vi "GDSString_FromatedTextToHTML.vi"(8 "error in (no error)":errorcluster, 11 "FormattedStringIn":refnum<vi>) -> (0 "error out":errorcluster, 2 "TextOut":string="<B</<1700FF<I</000000</I>>>>B>>ABCD", 3 "FormattedStringOut":refnum<vi>)   [LabVIEW 2020]
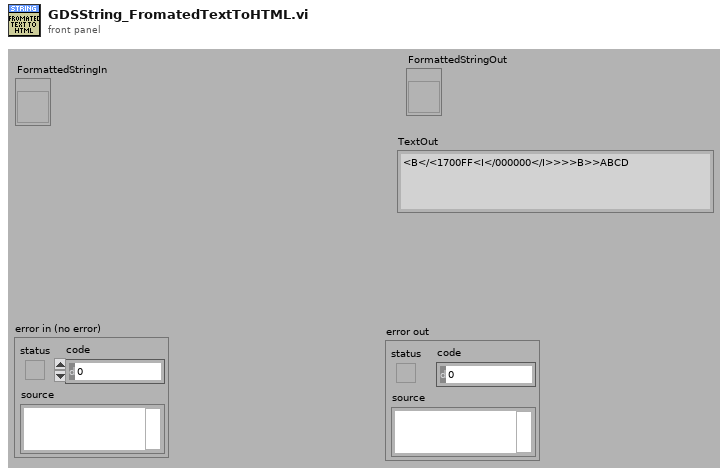
[diagram p1: front panel]
types:
  T1 = cluster{"i":i32, "Start":bool, "Type":enum16{"B", "I", "U", "C"}, "Data":variant}[]
  T2 = cluster{"i":i32, "Start":bool, "Type":enum16{"B", "I", "U", "C"}, "Data":variant}
  T3 = typedef "LVFontTypeDef.ctl" = cluster{"Font Name":string, "Size":u16, "Bold":bool, "Italic":bool, "Underline":bool, "Strikeout":bool, "Color":u32}
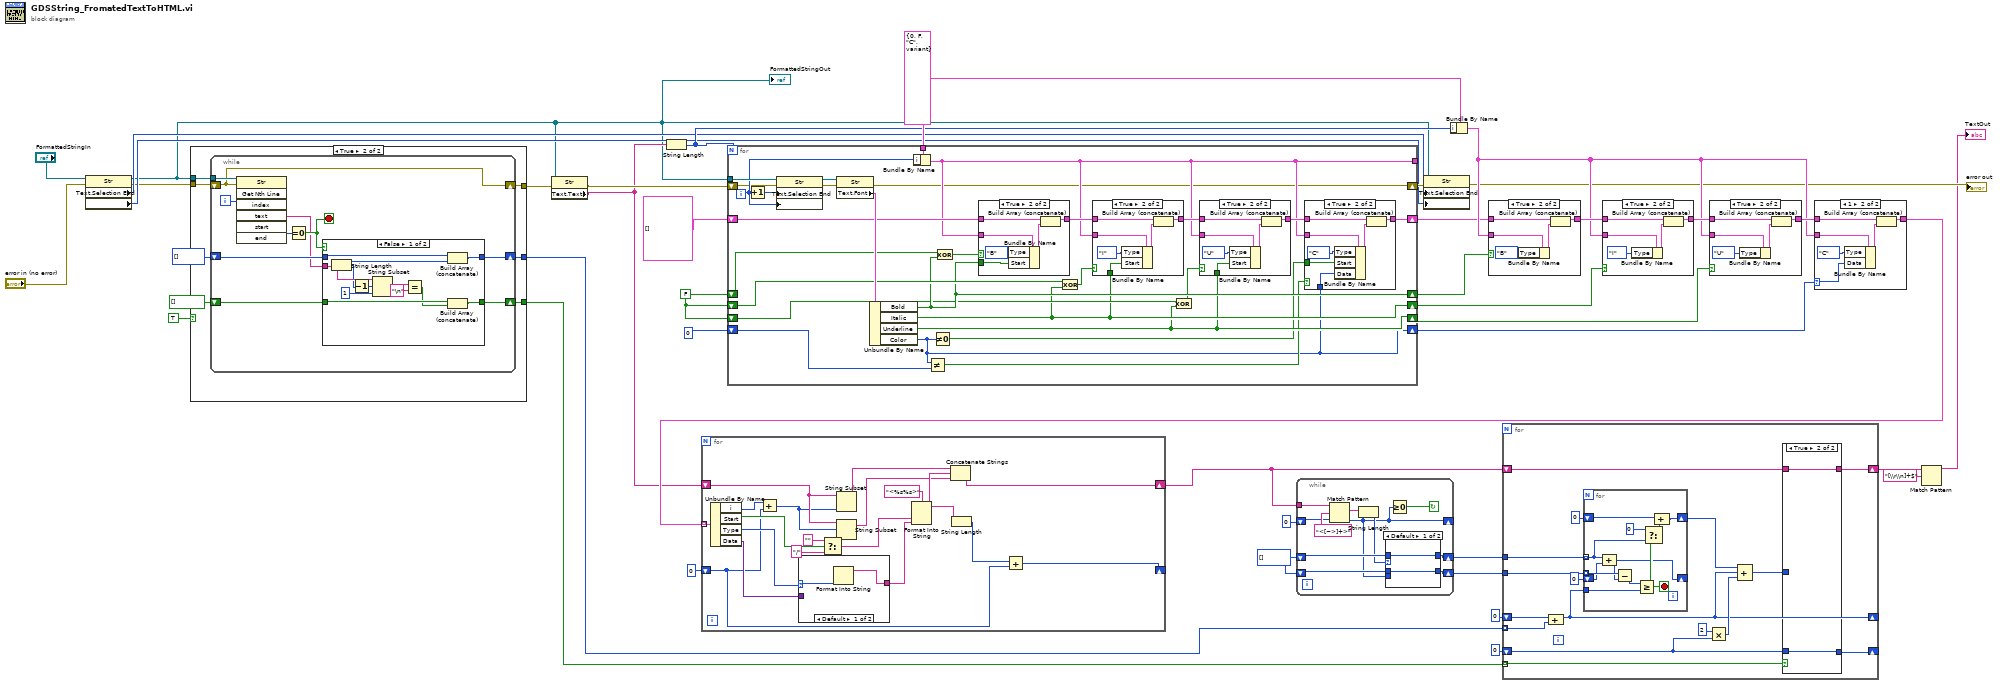
[diagram p0: block diagram]
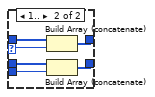
[diagram p2: hidden frame]
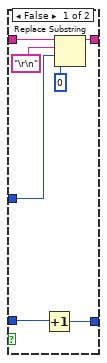
[diagram p3: hidden frame]
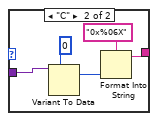
[diagram p10: hidden frame]
diagram:
  w11 = i32[] []
  w39 = FALSE ("Bold")
  w30 = T2 {"i"=0, "Start"=FALSE, "Type"=enum."C", "Data"=variant}
  n1 = property on="Property Node" class="Str"(reference="FormattedStringIn", error in="error in (no error)") -> (reference out=w13:refnum<vi>, error out=w17:errorcluster, "Text.Selection End"=w20:u32, "Text.Selection Start"=w19:u32)
  "FormattedStringOut" <- w13
  n2 = case shown="True" TRUE {
    tunnel: w13 -> [_ w48]
    tunnel: w17 -> [w41 w47]
    tunnel: [_ w45] -> w6
    tunnel: [w41 w46] -> w16
    tunnel: [_ w42] -> w2
    frame False {
    }
    frame True {
      n3 = while {
        tunnel: w48 -> [w57]
        shift-right: [w55] -> w45
        shift-left: i32[] [] -> [w54]
        shift-right: [w53] -> w46
        shift-left: w47 -> [w53]
        shift-right: [w51] -> w42
        shift-left: bool[] [] -> [w52]
        i -> [w58]
        stop <- w56 stop-if-true
        n4 = invoke on="Invoke Node" class="Str" method="Get Nth Line"(reference=w57, error in=w53, "index"=w58) -> ("text"=w50:string, "end"=w49:u32)  [unwired: 4 in, 5 out]
        n5 = Equal To 0?(x=w49) -> (x = 0?=w56:bool)
        n6 = case shown="False" w56 {
          tunnel: w50 -> [w65 _]
          tunnel: [w68 w71] -> w55
          tunnel: w54 -> [w69 w71]
          tunnel: [w67 w70] -> w51
          tunnel: w52 -> [w66 w70]
          frame False {
            n7 = String Length(string=w65) -> (length=w60:i32)
            n8 = Decrement(x=w60) -> (x-1=w63:i32)
            n9 = String Subset(string=w65, offset (0)=w63, length (rest)=1 ("length (rest)")) -> (substring=w62:string)
            n10 = Equal?(x=w62, y="\n") -> (x = y?=w59:bool)
            n11 = Build Array (concatenate)(w69, w60) -> (w68:i32[])
            n12 = Build Array (concatenate)(w66, w59) -> (w67:bool[])
          }
          frame True {
          }
        }
      }
    }
  }
  n13 = property class="Str"(reference=w13, error in=w16) -> (error out=w15:errorcluster, "Text.Text"=w14:string)  [unwired: 1 out]
  n14 = String Length(string=w14) -> (length=w29:i32)
  n15 = for {
    N: w29 -> [_]
    tunnel: w13 -> [w99]
    shift-right: [w90] -> w27
    shift-left: T1 [] -> [w95]
    tunnel: w30 -> [w94]
    shift-right: [w84] -> w34
    shift-left: w39 -> [w88]
    shift-right: [w81] -> w33
    shift-left: w39 -> [w85]
    shift-right: [w80] -> w32
    shift-left: w39 -> [w82]
    shift-right: [w76] -> w31
    shift-left: u32 0 ("Color") -> [w79]
    tunnel: [w75] -> _
    shift-right: [w72] -> w22
    shift-left: w15 -> [w74]
    i -> [w93]
    n16 = Increment(x=w93) -> (x+1=w97:i32)
    n17 = property class="Str"(reference=w99, error in=w74, "Text.Selection End"=w97, "Text.Selection Start"=w93) -> (reference out=w98:refnum<vi>, error out=w73:errorcluster)
    n18 = property class="Str"(reference=w98, error in=w73) -> (error out=w72:errorcluster, "Text.Font"=w96:T3)  [unwired: 1 out]
    n19 = Unbundle By Name(w96) -> ("Bold"=w84:bool, "Italic"=w81:bool, "Underline"=w80:bool, "Color"=w76:u32)
    n20 = Bundle By Name(cluster=w94, "i"=w93) -> (w75:T2)
    n21 = Not Equal?(x=w76, y=w79) -> (x != y?=w78:bool)
    n22 = Not Equal To 0?(x=w76) -> (x != 0?=w77:bool)
    n23 = Exclusive Or(1:w84, 2:w88) -> (0:w87:bool)
    n24 = case shown="True" w87 {
      tunnel: w95 -> [w122 w128]
      tunnel: [w122 w127] -> w92
      tunnel: w75 -> [_ w126]
      tunnel: w84 -> [_ w123]
      frame False {
      }
      frame True {
        n25 = Bundle By Name(cluster=w126, "Type"=enum16{"B", "I", "U", "C"}."B", "Start"=w123) -> (w125:T2)
        n26 = Build Array (concatenate)(w128, w125) -> (w127:T1)
      }
    }
    n27 = Exclusive Or(1:w81, 2:w85) -> (0:w86:bool)
    n28 = case shown="True" w86 {
      tunnel: w92 -> [w115 w121]
      tunnel: [w115 w120] -> w91
      tunnel: w75 -> [_ w119]
      tunnel: w81 -> [_ w116]
      frame False {
      }
      frame True {
        n29 = Bundle By Name(cluster=w119, "Type"=enum16{"B", "I", "U", "C"}."I", "Start"=w116) -> (w118:T2)
        n30 = Build Array (concatenate)(w121, w118) -> (w120:T1)
      }
    }
    n31 = Exclusive Or(1:w80, 2:w82) -> (0:w83:bool)
    n32 = case shown="True" w83 {
      tunnel: w91 -> [w108 w114]
      tunnel: [w108 w113] -> w89
      tunnel: w75 -> [_ w112]
      tunnel: w80 -> [_ w109]
      frame False {
      }
      frame True {
        n33 = Bundle By Name(cluster=w112, "Type"=enum16{"B", "I", "U", "C"}."U", "Start"=w109) -> (w111:T2)
        n34 = Build Array (concatenate)(w114, w111) -> (w113:T1)
      }
    }
    n35 = case shown="True" w78 {
      tunnel: w89 -> [w100 w107]
      tunnel: [w100 w106] -> w90
      tunnel: w75 -> [_ w105]
      tunnel: w76 -> [_ w102]
      tunnel: w77 -> [_ w101]
      frame False {
      }
      frame True {
        n36 = Bundle By Name(cluster=w105, "Type"=enum16{"B", "I", "U", "C"}."C", "Start"=w101, "Data"=w102) -> (w104:T2)
        n37 = Build Array (concatenate)(w107, w104) -> (w106:T1)
      }
    }
  }
  n38 = property on="Property Node" class="Str"(reference=w13, error in=w22, "Text.Selection End"=w20, "Text.Selection Start"=w19) -> (error out=→"error out":errorcluster)  [unwired: 1 out]
  n39 = Bundle By Name(cluster=w30, "i"=w29) -> (w28:T2)
  n40 = case shown="True" w34 {
    tunnel: w27 -> [w129 w134]
    tunnel: [w129 w133] -> w35
    tunnel: w28 -> [_ w132]
    frame False {
    }
    frame True {
      n41 = Bundle By Name(cluster=w132, "Type"=enum16{"B", "I", "U", "C"}."B") -> (w131:T2)
      n42 = Build Array (concatenate)(w134, w131) -> (w133:T1)
    }
  }
  n43 = case shown="True" w33 {
    tunnel: w35 -> [w135 w140]
    tunnel: [w135 w139] -> w36
    tunnel: w28 -> [_ w138]
    frame False {
    }
    frame True {
      n44 = Bundle By Name(cluster=w138, "Type"=enum16{"B", "I", "U", "C"}."I") -> (w137:T2)
      n45 = Build Array (concatenate)(w140, w137) -> (w139:T1)
    }
  }
  n46 = case shown="True" w32 {
    tunnel: w36 -> [w141 w146]
    tunnel: [w141 w145] -> w37
    tunnel: w28 -> [_ w144]
    frame False {
    }
    frame True {
      n47 = Bundle By Name(cluster=w144, "Type"=enum16{"B", "I", "U", "C"}."U") -> (w143:T2)
      n48 = Build Array (concatenate)(w146, w143) -> (w145:T1)
    }
  }
  n49 = case shown="1" w31 {
    selector: w31 -> [_ w148]
    tunnel: w37 -> [w147 w153]
    tunnel: [w147 w152] -> w26
    tunnel: w28 -> [_ w151]
    frame 0, Default {
    }
    frame 1 {
      n50 = Bundle By Name(cluster=w151, "Type"=enum16{"B", "I", "U", "C"}."C", "Data"=w148) -> (w150:T2)
      n51 = Build Array (concatenate)(w153, w150) -> (w152:T1)
    }
  }
  n52 = for {
    shift-right: [w155] -> w7
    shift-left: w14 -> [w165]
    tunnel: w26 -> [w172] mode=indexing
    shift-right: [w162] -> _
    shift-left: 0 -> [w160]
    n53 = Unbundle By Name(w172) -> ("i"=w161:i32, "Start"=w170:bool, "Type"=w167:enum16{"B", "I", "U", "C"}, "Data"=w166:variant)
    n54 = Add(x=w161, y=w160) -> (x+y=w159:i32)
    n55 = case shown="Default" w167 {
      selector: w167 -> [w174 _]
      tunnel: [w173 w175] -> w164
      tunnel: w166 -> [_ w179]
      frame Default {
        n56 = Format Into String(w174) -> (resulting string=w173:string)  [unwired: 3 in, 1 out]
      }
      frame "C" {
        n57 = Variant To Data(type=u32 0 ("Color"), Variant=w179) -> (data=w177:u32)  [unwired: 1 in, 1 out]
        n58 = Format Into String(format string="0x%06X", w177) -> (resulting string=w175:string)  [unwired: 2 in, 1 out]
      }
    }
    n59 = Select(t="", s=w170, f="/" ("format string")) -> (s? t:f=w163:string)
    n60 = String Subset(string=w165, length (rest)=w159) -> (substring=w158:string)  [unwired: 1 out]
    n61 = String Subset(string=w165, offset (0)=w159) -> (substring=w156:string)  [unwired: 1 out]
    n62 = Format Into String(format string="<%s%s>", w163, w164) -> (resulting string=w157:string)  [unwired: 2 in, 1 out]
    n63 = Concatenate Strings(w158, w157, w156) -> (w155:string)
    n64 = String Length(string=w157) -> (length=w154:i32)
    n65 = Add(x=w154, y=w160) -> (x+y=w162:i32)
  }
  n66 = while {
    shift-right: [w188] -> w10
    shift-left: w11 -> [w189]
    tunnel: w7 -> [w187]
    shift-right: [w180] -> _
    shift-left: 0 ("offset past match") -> [w186]
    shift-right: [w182] -> w9
    shift-left: w11 -> [w181]
    stop <- w184 continue-if-true
    n67 = Match Pattern(string=w187, regular expression="<[~>]+>", offset (0)=w186) -> (match substring=w185:string, offset past match=w180:i32)  [unwired: 2 out]
    n68 = String Length(string=w185) -> (length=w183:i32)
    n69 = case shown="Default" w183 {
      selector: w183 -> [_ w196]
      tunnel: w189 -> [w192 w198]
      tunnel: [w192 w197] -> w188
      tunnel: w181 -> [w191 w194]
      tunnel: [w191 w195] -> w182
      tunnel: w180 -> [_ w193]
      frame Default {
      }
      frame 1.. {
        n70 = Build Array (concatenate)(w198, w196) -> (w197:i32[])
        n71 = Build Array (concatenate)(w194, w193) -> (w195:i32[])
      }
    }
    n72 = Greater Or Equal To 0?(x=w180) -> (x >= 0?=w184:bool)
  }
  n73 = for {
    tunnel: w6 -> [w209] mode=indexing
    shift-right: [w214] -> w5
    shift-left: w7 -> [w213]
    tunnel: w10 -> [w205]
    tunnel: w9 -> [w210]
    shift-right: [w203] -> _
    shift-left: 0 -> [w211]
    tunnel: w2 -> [w199] mode=indexing
    shift-right: [w201] -> _
    shift-left: 0 -> [w202]
    n74 = Compound Arithmetic op=ADD(w211, w209) -> (w203:i32)
    n75 = for {
      tunnel: w210 -> [w228] mode=indexing
      tunnel: w203 -> [w234]
      tunnel: w205 -> [w227] mode=indexing
      shift-right: [w229] -> w206
      shift-left: 0 ("length (len. of substring)") -> [w230]
      shift-right: [w224] -> _
      shift-left: 0 ("length (len. of substring)") -> [w226]
      stop <- w233 stop-if-true
      n76 = Compound Arithmetic op=ADD(w227, w226) -> (w224:i32)
      n77 = Subtract(x=w228, y=w224) -> (x-y=w225:i32)
      n78 = Greater Or Equal?(x=w225, y=w234) -> (x >= y?=w233:bool)
      n79 = Select(t=0 ("length (len. of substring)"), s=w233, f=w227) -> (s? t:f=w231:i32)
      n80 = Compound Arithmetic op=ADD(w230, w231) -> (w229:i32)
    }
    n81 = Multiply(x=2 ("y"), y=w202) -> (x*y=w208:i32)
    n82 = Compound Arithmetic op=ADD(w206, w203, w208) -> (w207:i32)
    n83 = case shown="True" w199 {
      tunnel: [w221 w222] -> w214
      tunnel: w213 -> [w219 w222]
      tunnel: w207 -> [w218 _]
      tunnel: w202 -> [w216 w223]
      tunnel: [w215 w223] -> w201
      frame False {
        n84 = Increment(x=w216) -> (x+1=w215:i32)
        n85 = Replace Substring(2:0 ("length (len. of substring)"), 3:w218, 4:"\r\n" ("substring (\"\")"), 5:w219) -> (1:w221:string)  [unwired: 1 out]
      }
      frame True {
      }
    }
  }
  n86 = Match Pattern(string=w5, regular expression="[\\r\\n]+$") -> (before substring=→"TextOut":string)  [unwired: 1 in, 3 out]
